vi "Validate File Name Format.vi"(8 "error in":errorcluster, 11 "name format in":string) -> (0 "error out":errorcluster, 3 "name format out":string)   [LabVIEW 2018, in "GLog.lvlib" / "File Handler.lvclass"]
uses:
  File Handler.lvclass
  dependencies/Utilities/Utilities.lvlib
panel:
  # "Connector Pane"
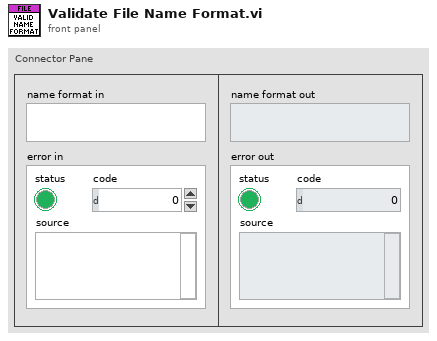
[diagram p1: front panel]
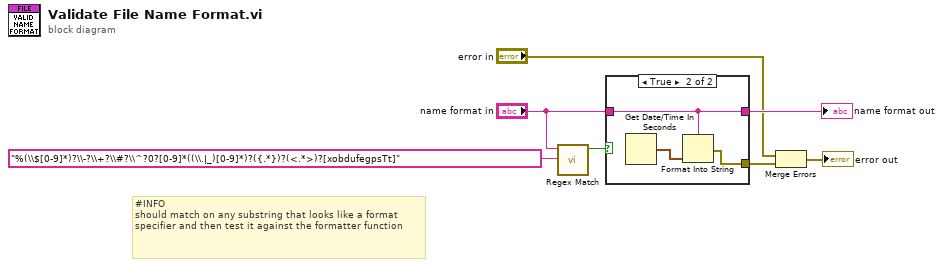
[diagram p0: block diagram]
diagram:
  # "#INFO\nshould match on any substring that looks like a format specifier and then test it against the formatter function"
  n1 = call "Regex Match.vi"("regular expression"="%(\\$[0-9]*)?\\-?\\+?\\#?\\^?0?[0-9]*((\\.|_)[0-9]*)?({.*})?(<.*>)?[xobdufegpsTt]", "string"="name format in") -> ("match?"=w5:bool)  [unwired: 9 in]
  n2 = case shown="True" w5 {
    tunnel: [w8 w11] -> w7
    tunnel: "name format in" -> [w8 w11]
    tunnel: [_ w9] -> w3
    frame False {
    }
    frame True {
      n3 = Get Date/Time In Seconds() -> (seconds since 1Jan1904=w10:timestamp)
      n4 = Format Into String(format string=w11, w10) -> (error out=w9:errorcluster)  [unwired: 2 in, 1 out]
    }
  }
  "name format out" <- w7
  n5 = Merge Errors("error in", w3) -> (→"error out":errorcluster)
